vi "Divide Test Items.vi"(11 "Test Item Name":string[](array[string])=["SDD21", "SDD22", "SCD21", "SCD22", "SCC11", "SCC22", "NEXT", "FEXT"]) -> (1 "Crosstalk  Item List":string[](array[string]), 3 "S-Para Item List":string[](array[string]))   [LabVIEW 2011]
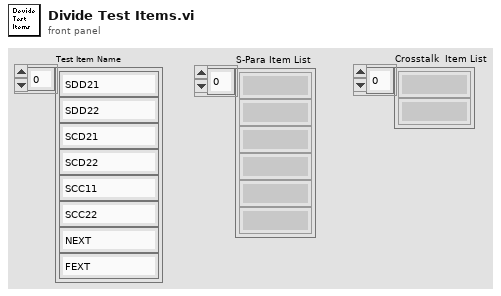
[diagram p1: front panel]
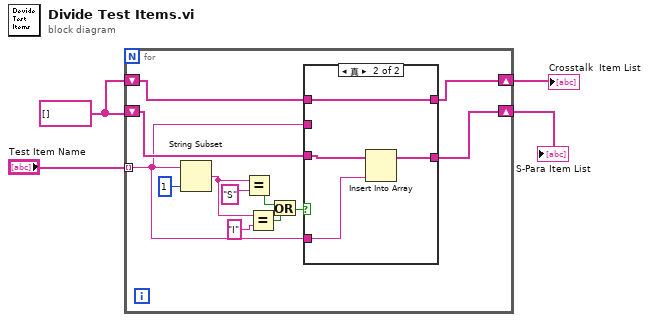
[diagram p0: block diagram]
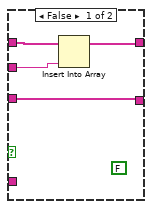
[diagram p2: hidden frame]
diagram:
  w2 = string[] []
  n1 = for {
    tunnel: "Test Item Name" -> [w10] mode=indexing
    shift-right: [w13] -> w3
    shift-left: w2 -> [w14]
    shift-right: [w11] -> w1
    shift-left: w2 -> [w12]
    n2 = String Subset(string=w10, length (rest)=1 ("长度（剩余）")) -> (substring=w9:string)  [unwired: 1 in]
    n3 = Equal?(x=w9, y="S") -> (x = y?=w8:bool)
    n4 = Equal?(x=w9, y="I") -> (x = y?=w7:bool)
    n5 = Or(x=w8, y=w7) -> (x .or. y?=w6:bool)
    n6 = case shown="真" w6 {
      tunnel: w14 -> [w20 w24]
      tunnel: w10 -> [_ w23]
      tunnel: [w20 w22] -> w13
      tunnel: w12 -> [w19 w21]
      tunnel: [w17 w21] -> w11
      tunnel: w10 -> [w18 _]
      frame False {
        (unwired) FALSE
        n7 = Insert Into Array(array=w19, new element=w18) -> (w17:string[])  [unwired: 1 in]
      }
      frame True {
        n8 = Insert Into Array(array=w24, new element=w23) -> (w22:string[])  [unwired: 1 in]
      }
    }
  }
  "S-Para Item List" <- w3
  "Crosstalk  Item List" <- w1
